vi "Pracownia4.2.vi"() -> ()   [LabVIEW 2019]
panel:
  out "Rozmiar tablicy":i32[](array[numeric])
  out "Suma":dbl
  out "Indeks maks.":i32[](array[numeric])
  out "Indeks min":i32[](array[numeric])
  out "Wartość maks.":dbl
  out "Wartość min.":dbl
  in  "?":bool
  out "Tablica wyjściowa":dbl[][](array[numeric])
  in  "Indeks Kolumny":dbl
  in  "Indeks wiersza":dbl
  in  "Wypełnianie \ntablicy wstawianej":dbl
  out "Tablica wstawiania":dbl[][](array[numeric])
  in  "Wprowadzanie danych":dbl[][](array[numeric])
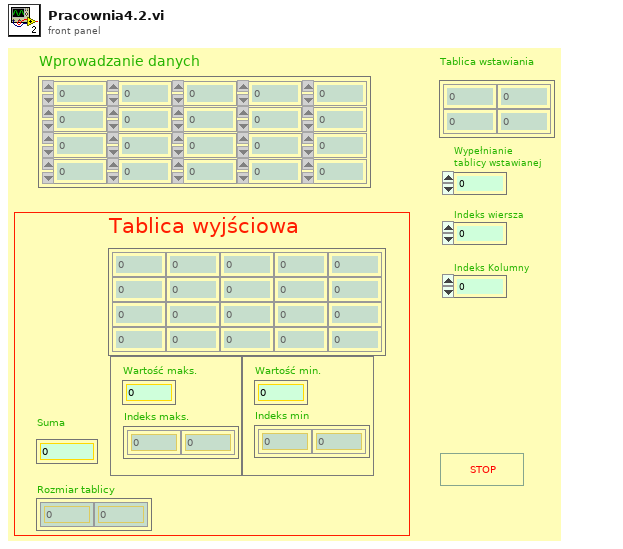
[diagram p1: front panel]
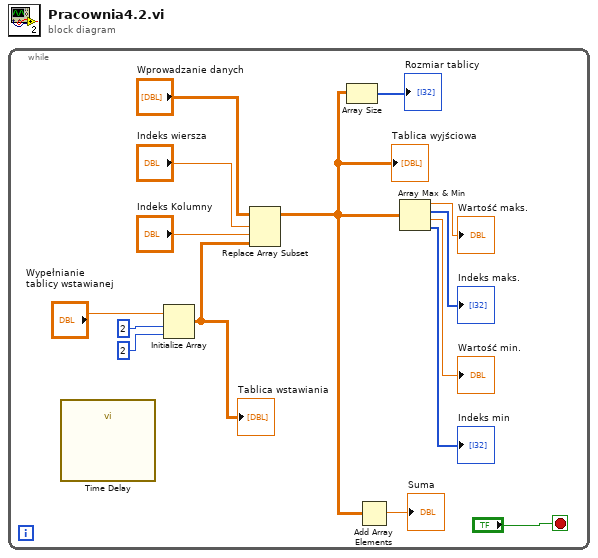
[diagram p0: block diagram]
diagram:
  n1 = while {
    stop <- "?" stop-if-true
    n2 = call "Time Delay"() -> ()  [unwired: 11 in, 1 out]
    n3 = Initialize Array("Wypełnianie \ntablicy wstawianej", 2 ("dimension size"), 2 ("dimension size")) -> (w1:dbl[][])
    "Tablica wstawiania" <- w1
    n4 = Replace Array Subset(array="Wprowadzanie danych", new element=w1, index (row)="Indeks wiersza", index (col)="Indeks Kolumny") -> (w3:dbl[][])
    "Tablica wyjściowa" <- w3
    n5 = Array Size(array=w3) -> (size(s)=→"Rozmiar tablicy":i32[])
    n6 = Add Array Elements(numeric array=w3) -> (sum=→"Suma":dbl)
    n7 = Array Max & Min(array=w3) -> (max value=→"Wartość maks.":dbl, max index (indices)=→"Indeks maks.":i32[], min value=→"Wartość min.":dbl, min index (indices)=→"Indeks min":i32[])
  }
